vi "Logfile Paths.vi"(11 "File Name":string) -> (1 "Alarm CSV Logfile path":path, 2 "TDMS Logfile path":path, 3 "CSV Logfile path":path)   [LabVIEW 2018, in "Waveform Loop.lvlib"]
uses:
  Waveform Loop.lvlib
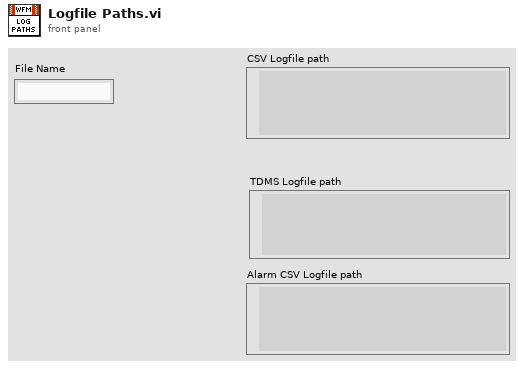
[diagram p1: front panel]
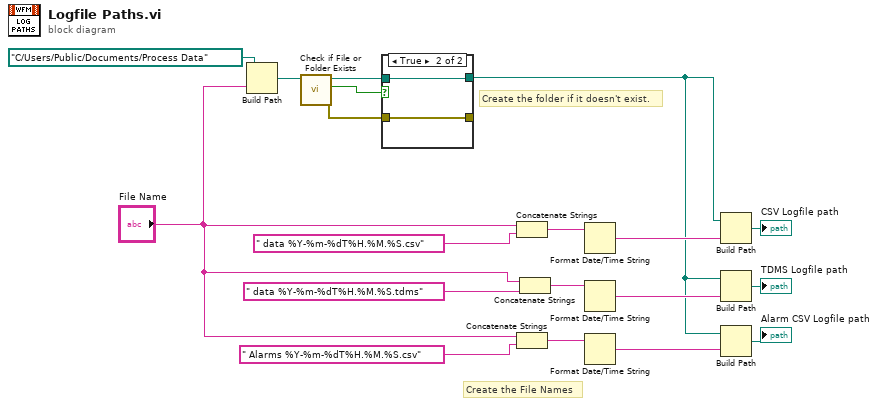
[diagram p0: block diagram]
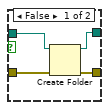
[diagram p2: hidden frame]
diagram:
  # "Create the folder if it doesn't exist."
  # "Create the File Names"
  n1 = Build Path(base path=path "C:/Users/Public/Documents/Process Data" ("Path"), name or relative path="File Name") -> (appended path=w5:path)
  n2 = call <vilib>:"Check if File or Folder Exists.vi"("path"=w5) -> ("error out"=w3:errorcluster, "file or folder exists?"=w2:bool, "dup path"=w1:path)  [unwired: 8 in]
  n3 = case shown="True" w2 {
    tunnel: w1 -> [w23 w24]
    tunnel: w3 -> [w22 w25]
    tunnel: [w21 w25] -> _
    tunnel: [w20 w24] -> w6
    frame False {
      n4 = Create Folder(path (use dialog)=w23, error in=w22) -> (created path=w20:path, error out=w21:errorcluster)  [unwired: 1 in, 1 out]
    }
    frame True {
    }
  }
  n5 = Concatenate Strings("File Name", " data %Y-%m-%dT%H.%M.%S.csv" ("time format string (%c)")) -> (w13:string)
  n6 = Concatenate Strings("File Name", " Alarms %Y-%m-%dT%H.%M.%S.csv" ("time format string (%c)")) -> (w11:string)
  n7 = Concatenate Strings("File Name", " data %Y-%m-%dT%H.%M.%S.tdms" ("time format string (%c)")) -> (w12:string)
  n8 = Format Date/Time String(time format string (%c)=w13) -> (date/time string=w19:string)  [unwired: 2 in]
  n9 = Format Date/Time String(time format string (%c)=w12) -> (date/time string=w16:string)  [unwired: 2 in]
  n10 = Format Date/Time String(time format string (%c)=w11) -> (date/time string=w9:string)  [unwired: 2 in]
  n11 = Build Path(base path=w6, name or relative path=w19) -> (appended path=→"CSV Logfile path":path)
  n12 = Build Path(base path=w6, name or relative path=w16) -> (appended path=→"TDMS Logfile path":path)
  n13 = Build Path(base path=w6, name or relative path=w9) -> (appended path=→"Alarm CSV Logfile path":path)
